vi "notificadores.vi"() -> ()   [LabVIEW 2016]
panel:
  out "error out":errorcluster
  in  "espera 2":u32
  out "indice 2":i32
  out "Waveform Chart 2":dbl(graph)
  out "Waveform Chart":dbl(graph)
  out "indice 1":i32
  in  "espera 1":u32
  in  "B1":bool
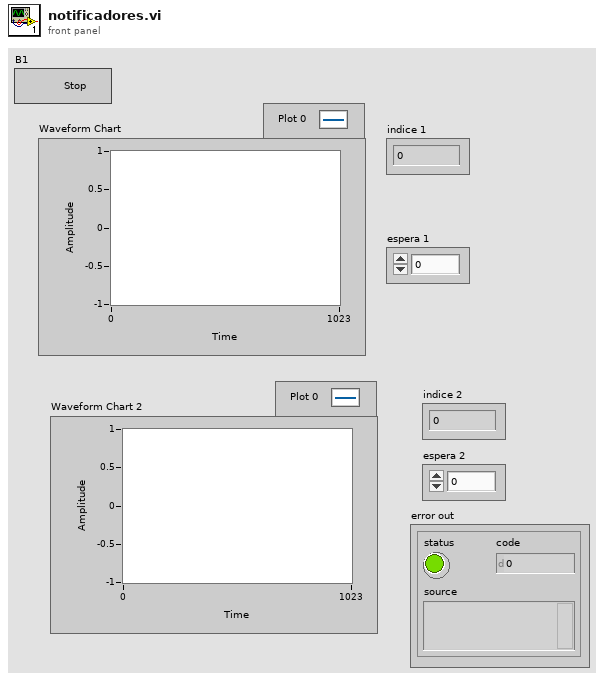
[diagram p1: front panel]
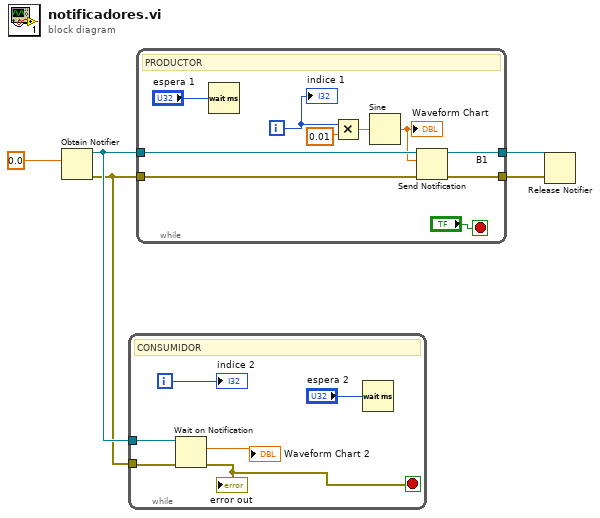
[diagram p0: block diagram]
diagram:
  n1 = Obtain Notifier(notification data type=0.0) -> (notifier out=w5:refnum<notifier>, error out=w4:errorcluster)  [unwired: 3 in, 1 out]
  n2 = while {
    tunnel: w5 -> [w9]
    tunnel: w4 -> [w8]
    i -> [w10]
    stop <- w6 stop-if-true
    # "CONSUMIDOR"
    n3 = Wait on Notification(notifier=w9, error in (no error)=w8) -> (notification=→"Waveform Chart 2":dbl, error out=w6:errorcluster)  [unwired: 2 in, 2 out]
    "error out" <- w6
    n4 = Wait (ms)(milliseconds to wait="espera 2") -> ()  [unwired: 1 out]
    "indice 2" <- w10
  }
  n5 = while {
    tunnel: w5 -> [w16]
    tunnel: w4 -> [w15]
    tunnel: [w14] -> w2
    tunnel: [w13] -> w1
    i -> [w19]
    stop <- "B1" stop-if-true
    # "PRODUCTOR"
    n6 = Wait (ms)(milliseconds to wait="espera 1") -> ()  [unwired: 1 out]
    n7 = Multiply(x=w19, y=0.01) -> (x*y=w18:dbl)
    n8 = Sine(x=w18) -> (sin(x)=w12:dbl)
    "Waveform Chart" <- w12
    n9 = Send Notification(notification=w12, notifier=w16, error in (no error)=w15) -> (notifier out=w14:refnum<notifier>, error out=w13:errorcluster)
    "indice 1" <- w19
  }
  n10 = Release Notifier(notifier=w2, error in (no error)=w1) -> ()  [unwired: 1 in, 3 out]
